vi "Create Sync Frame & Session.vi"(8 "error in (no error)":errorcluster, 9 "Interface Name":string, 10 "Sync Packet Name":string, 11 "XNET Database Ref":refnum<k21>) -> (0 "error out":errorcluster, 3 "Dummy XNET Session":refnum<k21>)   [LabVIEW 2013, in "Trigger Timestamp Logging Engine.lvlib"]
uses:
  Trigger Timestamp Logging Engine.lvlib
  <vilib>/xnet/xnet.llb/XNET Database Create (Frame).vi
  <vilib>/xnet/xnet.llb/XNET Create Session (Frame Input Single-point).vi
  <vilib>/xnet/xnet.llb/XNET Database Close (Database).vi
  <resource>/objmgr/xnet.rc
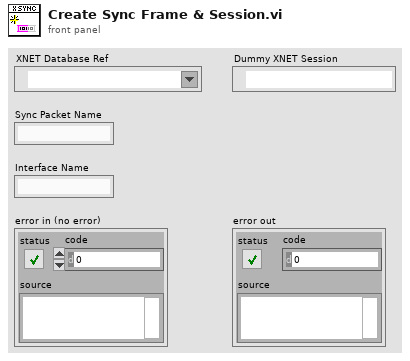
[diagram p1: front panel]
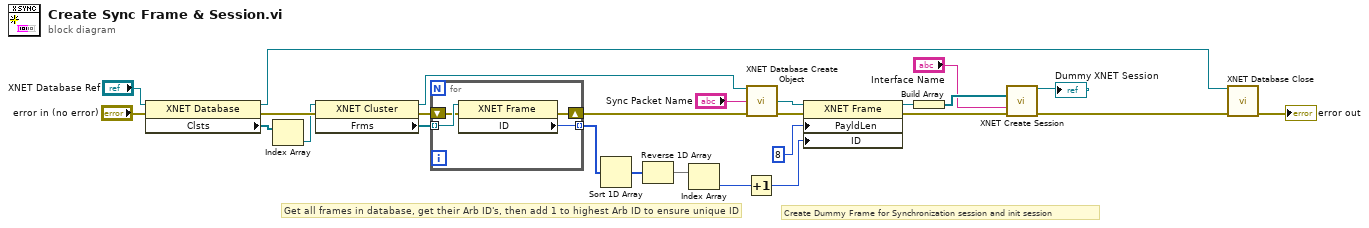
[diagram p0: block diagram]
diagram:
  # "Create Dummy Frame for Synchronization session and init session"
  # "Get all frames in database, get their Arb ID's, then add 1 to highest Arb ID to ensure unique ID"
  n1 = property class="XNET Database"(reference="XNET Database Ref", error in="error in (no error)") -> (reference out=w24:refnum<k21>, error out=w7:errorcluster, "Clsts"=w2:refnum<k21>[])
  n2 = Index Array(array=w2) -> (element=w1:refnum<k21>)  [unwired: 1 in]
  n3 = property class="XNET Cluster"(reference=w1, error in=w7) -> (reference out=w14:refnum<k21>, error out=w8:errorcluster, "Frms"=w9:refnum<k21>[])
  n4 = for {
    tunnel: w9 -> [w30] mode=indexing
    tunnel: [w29] -> w10 mode=indexing
    shift-right: [w27] -> w15
    shift-left: w8 -> [w28]
    n5 = property class="XNET Frame"(reference=w30, error in=w28) -> (error out=w27:errorcluster, "ID"=w29:u32)  [unwired: 1 out]
  }
  n6 = Sort 1D Array(array=w10) -> (sorted array=w11:u32[])
  n7 = Reverse 1D Array(array=w11) -> (reversed array=w12:u32[])
  n8 = Index Array(array=w12) -> (element=w13:u32)  [unwired: 1 in]
  n9 = Increment(x=w13) -> (x+1=w20:u32)
  n10 = call-poly <vilib>:"XNET Database Create Object.vi"("cluster in"=w14, "frame name"="Sync Packet Name", "error in (no error)"=w15) -> ("frame out"=w17:refnum<k21>, "error out"=w18:errorcluster)  [unwired: 10 in, 1 out]
  n11 = property class="XNET Frame"(reference=w17, error in=w18, "PayldLen"=u32 8 ("Payload Length"), "ID"=w20) -> (reference out=w21:refnum<k21>, error out=w23:errorcluster)
  n12 = Build Array(w21) -> (w22:refnum<k21>[])
  n13 = call-poly <vilib>:"XNET Create Session.vi"("frame list"=w22, "interface"="Interface Name", "error in (no error)"=w23) -> ("session out"=→"Dummy XNET Session":refnum<k21>, "error out"=w25:errorcluster)  [unwired: 11 out]
  n14 = call-poly <vilib>:"XNET Database Close.vi"("database in"=w24, "error in (no error)"=w25) -> ("error out"=→"error out":errorcluster)  [unwired: 13 in]
